vi "Pre Launch Init.vi"(11 "First Actor in":refnum<class "First Actor.lvclass">) -> (0 "error out":errorcluster, 3 "First Actor out":refnum<class "First Actor.lvclass">)   [LabVIEW 2021, in "First Actor.lvlib" / "First Actor.lvclass"]
doc: "(<B>Filename</B>: Actor Framework.lvlib:Actor.lvclass:Pre Launch Init.vi)\n\nDefines behavior that occurs after the Launch Nested Actor method is invoked but before the actor's Actor Core method begins running.\n\nBy default, this method does nothing. A descendant class may override it to define behavior."
uses:
  First Actor.lvclass
  <vilib>/ActorFramework/Actor/Actor.lvclass
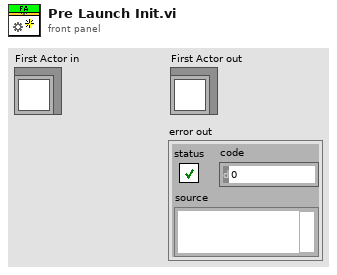
[diagram p1: front panel]
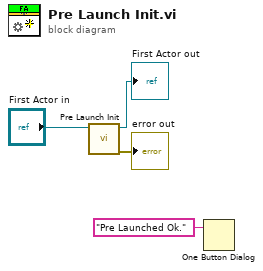
[diagram p0: block diagram]
diagram:
  n1 = call-parent "Pre Launch Init.vi"("Actor in"="First Actor in") -> ("error out"=→"error out":errorcluster, "Actor out"=→"First Actor out":refnum<class "First Actor.lvclass">)  [unwired: 9 in]
  n2 = One Button Dialog(message="Pre Launched Ok.") -> ()  [unwired: 1 in, 1 out]
